vi "Voltage to Color.vi"(11 "Array in":dbl[][](array[numeric])) -> (3 "Array out":u32[][](array[numeric]))   [LabVIEW 2016]
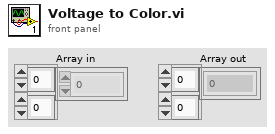
[diagram p1: front panel]
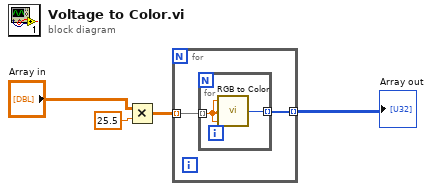
[diagram p0: block diagram]
diagram:
  n1 = Multiply(x="Array in", y=25.5) -> (x*y=w2:dbl[][])
  n2 = for {
    tunnel: w2 -> [w6] mode=indexing
    tunnel: [w5] -> w1 mode=indexing
    n3 = for {
      tunnel: w6 -> [w8] mode=indexing
      tunnel: [w7] -> w5 mode=indexing
      n4 = call <vilib>:"RGB to Color.vi"("B"=w8, "G"=w8, "R"=w8) -> ("Color"=w7:u32)
    }
  }
  "Array out" <- w1
